vi "Configure Carrier (Carrier Reference).vi"(0 "VISA resource name":refnum<visa-resource-name>, 1 "Auto Reference Carrier Number (T: Enable)":bool=TRUE, 2 "Auto Reference Carrier Frequency (T: Enable)":bool=TRUE, 3 "Auto Power Reference (T: Enable)":bool=TRUE, 5 "Device Mode (1: BTS)":i32(ring)=1 items=["BTS"=1, "MS"=2], 7 "Measurement Type (0: Total Power Reference)":i32(ring) items=["Total Power Reference", "PSD Reference"], 11 "error in (no error)":errorcluster, 12 "Manual Reference Carrier Number (1)":i32=1 format="%.0g", 13 "Manual Reference Carrier Frequency (1E+9Hz)":dbl=1000000000.0 format="%#.6g", 14 "Manual Power Reference(10 dBm)":dbl=10.0 format="%#.6g") -> (4 "VISA resource name out":refnum<visa-resource-name>, 15 "error out":errorcluster)   [LabVIEW 2018, in "Agilent MXA Series.lvlib"]
doc: "Configures the Carriers Reference settings under ACP measurement type."
uses:
  Agilent MXA Series.lvlib
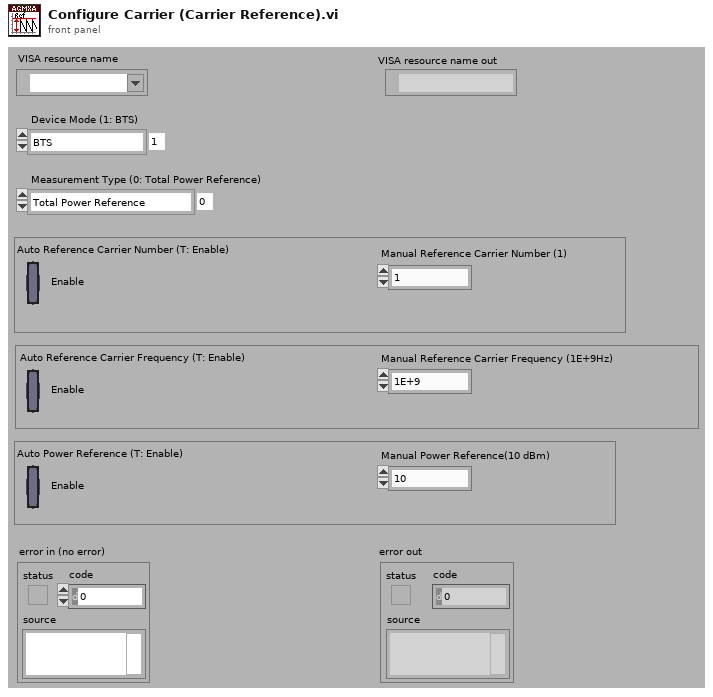
[diagram p1: front panel]
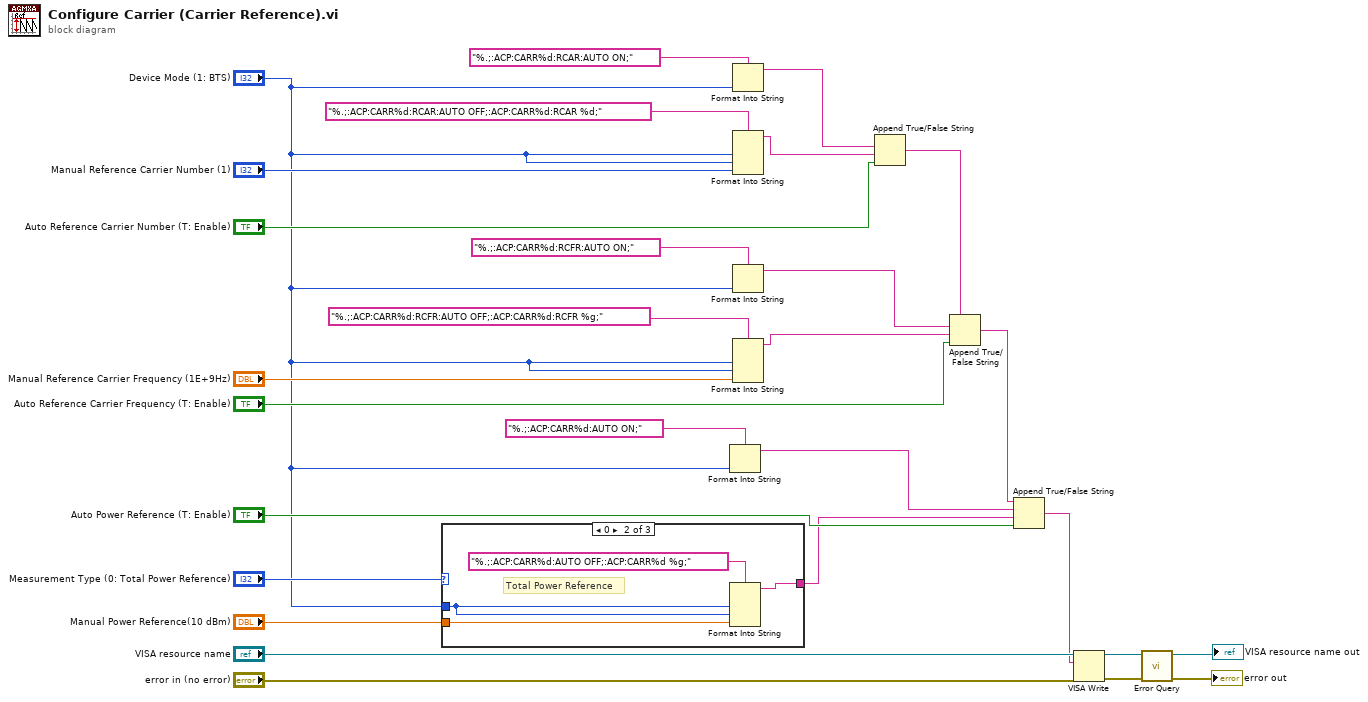
[diagram p0: block diagram]
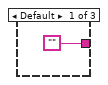
[diagram p2: hidden frame]
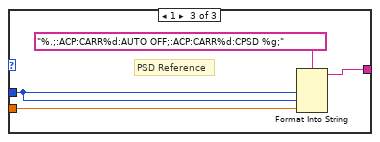
[diagram p3: hidden frame]
diagram:
  n1 = case shown="0" "Measurement Type (0: Total Power Reference)" {
    tunnel: "Device Mode (1: BTS)" -> [_ w31 w35]
    tunnel: "Manual Power Reference(10 dBm)" -> [_ w30 w34]
    tunnel: ["" w32 w36] -> w4
    frame Default {
    }
    frame 0 {
      # "Total Power Reference"
      n2 = Format Into String(format string="%.;:ACP:CARR%d:AUTO OFF;:ACP:CARR%d %g;", w31, w31, w30) -> (resulting string=w32:string)  [unwired: 2 in, 1 out]
    }
    frame 1 {
      # "PSD Reference"
      n3 = Format Into String(format string="%.;:ACP:CARR%d:AUTO OFF;:ACP:CARR%d:CPSD %g;", w35, w35, w34) -> (resulting string=w36:string)  [unwired: 2 in, 1 out]
    }
  }
  n4 = Format Into String(format string="%.;:ACP:CARR%d:AUTO ON;", "Device Mode (1: BTS)") -> (resulting string=w5:string)  [unwired: 2 in, 1 out]
  n5 = Format Into String(format string="%.;:ACP:CARR%d:RCAR:AUTO ON;", "Device Mode (1: BTS)") -> (resulting string=w24:string)  [unwired: 2 in, 1 out]
  n6 = Format Into String(format string="%.;:ACP:CARR%d:RCAR:AUTO OFF;:ACP:CARR%d:RCAR %d;", "Device Mode (1: BTS)", "Device Mode (1: BTS)", "Manual Reference Carrier Number (1)") -> (resulting string=w23:string)  [unwired: 2 in, 1 out]
  n7 = Format Into String(format string="%.;:ACP:CARR%d:RCFR:AUTO ON;", "Device Mode (1: BTS)") -> (resulting string=w18:string)  [unwired: 2 in, 1 out]
  n8 = Format Into String(format string="%.;:ACP:CARR%d:RCFR:AUTO OFF;:ACP:CARR%d:RCFR %g;", "Device Mode (1: BTS)", "Device Mode (1: BTS)", "Manual Reference Carrier Frequency (1E+9Hz)") -> (resulting string=w17:string)  [unwired: 2 in, 1 out]
  n9 = Append True/False String(1:"Auto Reference Carrier Number (T: Enable)", 2:w23, 3:w24) -> (0:w19:string)  [unwired: 1 in]
  n10 = Append True/False String(1:"Auto Reference Carrier Frequency (T: Enable)", 2:w17, 3:w18, 4:w19) -> (0:w2:string)
  n11 = Append True/False String(1:"Auto Power Reference (T: Enable)", 2:w4, 3:w5, 4:w2) -> (0:w1:string)
  n12 = VISA Write(VISA resource name="VISA resource name", write buffer=w1, error in (no error)="error in (no error)") -> (VISA resource name out=w10:refnum<visa-resource-name>, error out=w11:errorcluster)  [unwired: 1 out]
  n13 = call "Error Query.vi"("error in (no error)"=w11, "VISA resource name"=w10) -> ("error out"=→"error out":errorcluster, "VISA resource name out"=→"VISA resource name out":refnum<visa-resource-name>)  [unwired: 6 in, 2 out]
